vi "Area Computatio - Prompt user.vi"() -> ()   [LabVIEW 2020]
panel:
  out "output":dbl
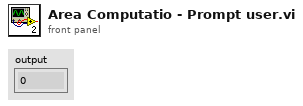
[diagram p1: front panel]
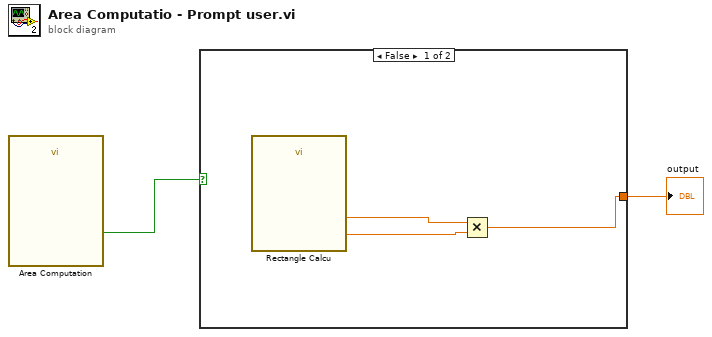
[diagram p0: block diagram]
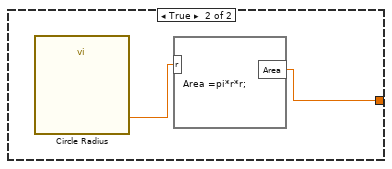
[diagram p2: hidden frame]
diagram:
  n1 = call "Area Computation"() -> ("Circle"=w2:bool)  [unwired: 16 in, 3 out]
  n2 = case shown="False" w2 {
    tunnel: [w3 w6] -> w1
    frame False {
      n3 = call "Rectangle Calcu"() -> ("Breadth"=w4:dbl, "Length"=w5:dbl)  [unwired: 16 in, 2 out]
      n4 = Multiply(x=w5, y=w4) -> (x*y=w3:dbl)
    }
    frame True {
      n5 = call "Circle Radius"() -> ("Radius"=w7:dbl)  [unwired: 17 in, 2 out]
      n6 = formula code="Area =pi*r*r;"("r"=w7) -> ("Area"=w6:dbl)
    }
  }
  "output" <- w1
